vi "WSVCAP SHL FPGA LL SPI FIFO Manager - Transfer.vi"(7 "timeout in ms (-1)":i32, 9 "Word In":u16, 11 "error in (no error)":errorcluster, 13 "Operation":T1) -> (4 "Data Out":u16, 8 "Timed Out":bool, 15 "error out":errorcluster)   [LabVIEW 2012]
uses:
  Type Defs/WSVCAP SHL FIFO Operation Enum.ctl
  <vilib>/rvi/DataTransferAndStorage/Container/XNode/niFpgaContainer.xnode
  <vilib>/rvi/FIFO/Fifo_Resource/nirvififoEmulationGetNumberOfElementsToRead.vi
  <vilib>/rvi/FIFO/Fifo_Resource/nirvififoEmulationWrite.vi
  <vilib>/rvi/FIFO/Fifo_Resource/nirvififoEmulationRead.vi
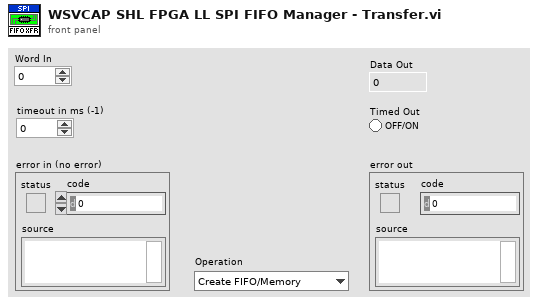
[diagram p1: front panel]
types:
  T1 = typedef "WSVCAP SHL FIFO Operation Enum.ctl" = enum16{"Create FIFO/Memory", "Get Write FIFO Status", "Get Read FIFO Status", "Put Element in Write", "Put Element in Read", "Get Element from Write", "Get Element from Read"}
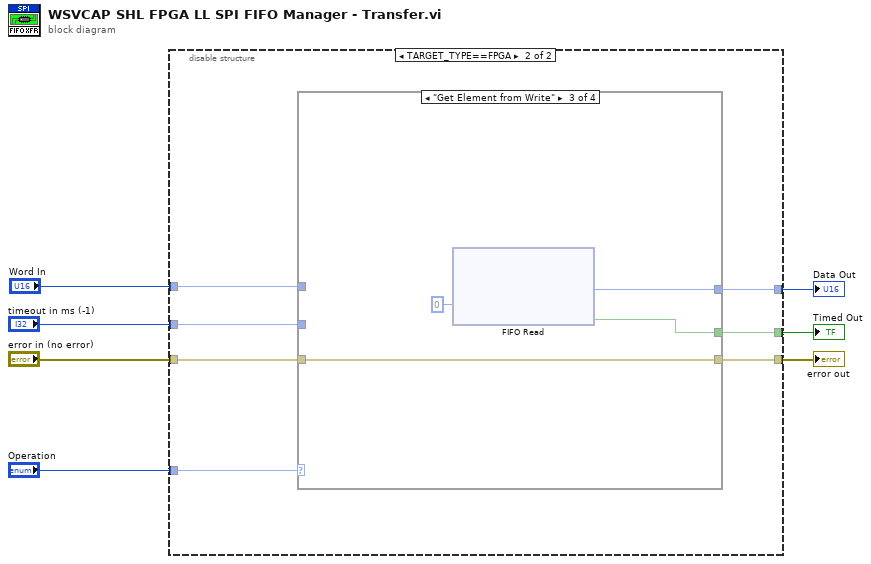
[diagram p0: block diagram]
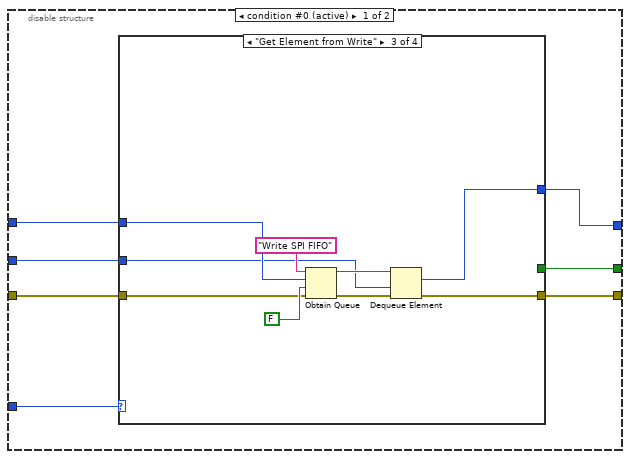
[diagram p2: hidden frame]
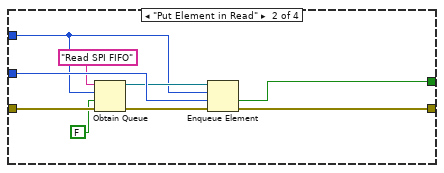
[diagram p4: hidden frame]
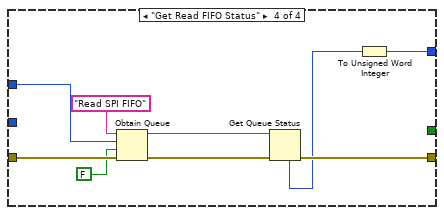
[diagram p5: hidden frame]
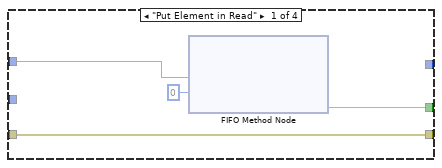
[diagram p6: hidden frame]
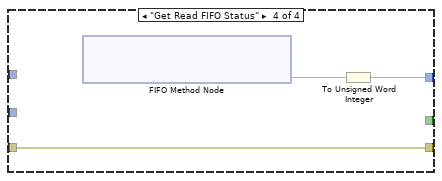
[diagram p8: hidden frame]
diagram:
  n1 = disable-structure shown="TARGET_TYPE==FPGA" {
    disable-tunnel: "Operation" -> [w14 w49]
    disable-tunnel: "error in (no error)" -> [w13 w46]
    disable-tunnel: [w12 w45] -> w5
    disable-tunnel: "timeout in ms (-1)" -> [w11 w48]
    disable-tunnel: [w10 w44] -> w1
    disable-tunnel: [w9 w47] -> w3
    disable-tunnel: "Word In" -> [w8 w43]
    frame condition #0 (active) {
      n2 = case shown="\"Get Element from Write\"" w14 {
        tunnel: [w15 w24 w28 w42] -> w12
        tunnel: w13 -> [w15 w21 w29 w41]
        tunnel: w11 -> [_ w23 w26 _]
        tunnel: [_ _ w25 w34] -> w10
        tunnel: [_ w22 _ _] -> w9
        tunnel: w8 -> [_ w16 w27 w38]
        frame Default {
        }
        frame "Put Element in Read" {
          n3 = Obtain Queue(name (unnamed)="Read SPI FIFO", element data type=w16, create if not found? (T)=FALSE, error in (no error)=w21) -> (queue out=w19:refnum<queue>, error out=w20:errorcluster)  [unwired: 1 in, 1 out]
          n4 = Enqueue Element(queue=w19, element=w16, timeout in ms (-1)=w23, error in (no error)=w20) -> (timed out?=w22:bool, error out=w24:errorcluster)  [unwired: 1 out]
        }
        frame "Get Element from Write" {
          n5 = Obtain Queue(name (unnamed)="Write SPI FIFO", element data type=w27, create if not found? (T)=FALSE, error in (no error)=w29) -> (queue out=w31:refnum<queue>, error out=w33:errorcluster)  [unwired: 1 in, 1 out]
          n6 = Dequeue Element(queue=w31, timeout in ms (-1)=w26, error in (no error)=w33) -> (element=w25:u16, error out=w28:errorcluster)  [unwired: 2 out]
        }
        frame "Get Read FIFO Status" {
          n7 = Obtain Queue(name (unnamed)="Read SPI FIFO", element data type=w38, create if not found? (T)=FALSE, error in (no error)=w41) -> (queue out=w37:refnum<queue>, error out=w36:errorcluster)  [unwired: 1 in, 1 out]
          n8 = Get Queue Status(queue=w37, error in (no error)=w36) -> (error out=w42:errorcluster, # elements in queue=w35:i32)  [unwired: 1 in, 6 out]
          n9 = To Unsigned Word Integer(number=w35) -> (unsigned 16bit integer=w34:u16)
        }
      }
    }
    frame condition #1 {
      n10 = case shown="\"Get Element from Write\"" w49 {
        tunnel: w48 -> [_ _ _ _]
        tunnel: [w52 _ w55 _] -> w47
        tunnel: w46 -> [w53 w54 w58 w59]
        tunnel: [w53 w54 w58 w59] -> w45
        tunnel: [_ _ w57 w60] -> w44
        tunnel: w43 -> [w50 _ _ _]
        frame "Put Element in Read" {
          n11 = xnode ("FIFO Method Node")("Element"=w50, "Timeout"=0) -> ("Timed Out?"=w52:bool)  [unwired: 2 in, 2 out]
        }
        frame Default {
        }
        frame "Get Element from Write" {
          n12 = xnode "FIFO Read"("Timeout"=0) -> ("Element"=w57:u16, "Timed Out?"=w55:bool)  [unwired: 1 in, 1 out]
        }
        frame "Get Read FIFO Status" {
          n13 = xnode ("FIFO Method Node")() -> ("Number of Elements to Read"=w61:u32)  [unwired: 2 in, 2 out]
          n14 = To Unsigned Word Integer(number=w61) -> (unsigned 16bit integer=w60:u16)
        }
      }
    }
  }
  "error out" <- w5
  "Timed Out" <- w3
  "Data Out" <- w1
